vi "DAQmx Create Channel (AI-Temperature-Thermocouple).vi"(0 "task in":refnum<k21>, 1 "maximum value":dbl=100.0 format="%0.2f", 2 "minimum value":dbl format="%0.2f", 5 "physical channels":tag, 6 "cjc source":i32(ring)=10116 items=["Built-In"=10200, "Constant Value"=10116, "Channel"=10113], 7 "name to assign":string, 9 "units":i32(ring)=10143 items=["Deg C"=10143, "Deg F"=10144, "Kelvins"=10325, "Deg R"=10145, "From Custom Scale"=10065], 10 "cjc channel":refnum<k21>, 11 "error in":errorcluster, 13 "thermocouple type":i32(ring)=10072 items=["J"=10072, "K"=10073, "N"=10077, "R"=10082, "S"=10085, "T"=10086, "B"=10047, "E"=10055], 14 "cjc value":dbl=25.0 format="%0.2f") -> (4 "task out":refnum<k21>, 15 "error out":errorcluster)   [LabVIEW 2011]
doc: "Creates channel(s) that use a thermocouple to measure temperature."
uses:
  C:/Program Files/National Instruments/LabVIEW 2011/resource/objmgr/daqmx.rc
panel:
  # "input limits"
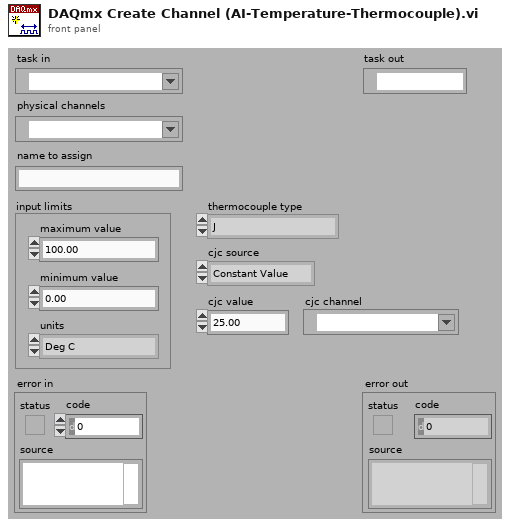
[diagram p1: front panel]
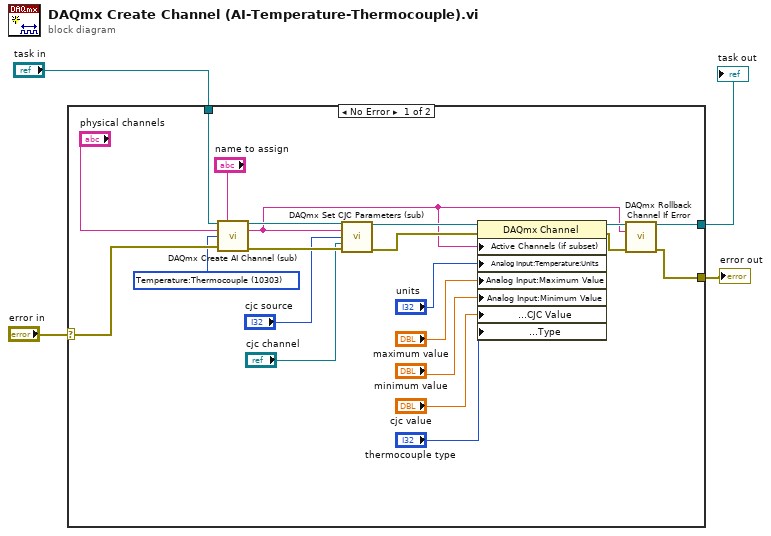
[diagram p0: block diagram]
diagram:
  n1 = case shown="No Error" "error in" {
    selector: "error in" -> [w24 w26]
    tunnel: [w6 w26] -> w4
    tunnel: "task in" -> [w25 w27]
    tunnel: [w7 w27] -> w1
    frame No Error {
      w17 = 10303 items=["Voltage"=10322, "Current"=10134, "More:Voltage:Custom with Excitation"=10323, "More:Current:Custom with Excitation"=10136, "Frequency"=10181, "Period"=10257, "Resistance"=10278, "Temperature:Thermocouple"=10303, "Temperature:Thermistor"=10302, "Temperature:RTD"=10301, "Temperature:Built-in Sensor"=10311, "Strain Gage"=10300] ("measurement type")
      n2 = call "DAQmx Create AI Channel (sub).vi"("task in"=w25, "virtual channel name"="name to assign", "physical channel name"="physical channels", "measurement type"=w17, "error in"=w24) -> ("task out"=w15:refnum<k21>, "channel names"=w5:string, "error out"=w14:errorcluster)  [unwired: 2 in, 6 out]
      n3 = call "DAQmx Set CJC Parameters (sub).vi"("task in"=w15, "thermocouple channel"=w5, "cjc source"="cjc source", "cjc channel"="cjc channel", "error in"=w14) -> ("task out"=w12:refnum<k21>, "error out"=w11:errorcluster)  [unwired: 9 out]
      n4 = property class="DAQmx Channel"(reference=w12, error in=w11, "Active Channels (if subset)"=w5, "Analog Input:Temperature:Units"="units", "Analog Input:Maximum Value"="maximum value", "Analog Input:Minimum Value"="minimum value", "Analog Input:Temperature:Thermocouple:CJC Value"="cjc value", "Analog Input:Temperature:Thermocouple:Type"="thermocouple type") -> (reference out=w9:refnum<k21>, error out=w8:errorcluster)
      n5 = call "DAQmx Rollback Channel If Error.vi"("task in"=w9, "channel names"=w5, "error in"=w8) -> ("task out"=w7:refnum<k21>, "error out"=w6:errorcluster)  [unwired: 11 out]
    }
    frame Error {
    }
  }
  "error out" <- w4
  "task out" <- w1
